vi "AngleStats_AngleAdd.vi"(6 "Row":i32, 10 "B":T1, 11 "A":T1) -> (3 "Result":T1)   [LabVIEW 2019, in "Trajectory_Library.lvlib"]
doc: "Creates a new LINEAR SYSTEM data cluster with the specified values. \n\n\nInputs: \n - XXX -- XXX.\n\nOutputs:\n - XXX -- XXX."
uses:
  <vilib>/Analysis/Matrix/Datatypes/RealMatrix.ctl
  MathUtil_InputModulus.vi
  Trajectory_Library.lvlib
  <vilib>/Analysis/Matrix/NI_Matrix.lvlib
  <vilib>/Analysis/Matrix/Numeric/Add/Add - RM,RM.vi
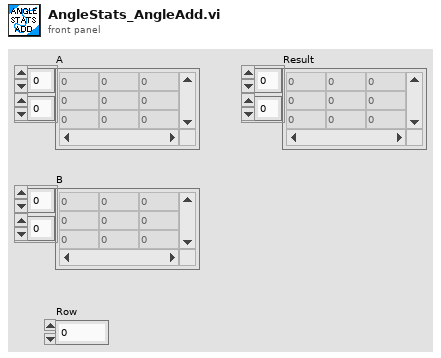
[diagram p1: front panel]
types:
  T1 = typedef "NI_Matrix.lvlib/RealMatrix.ctl" = dbl[][]
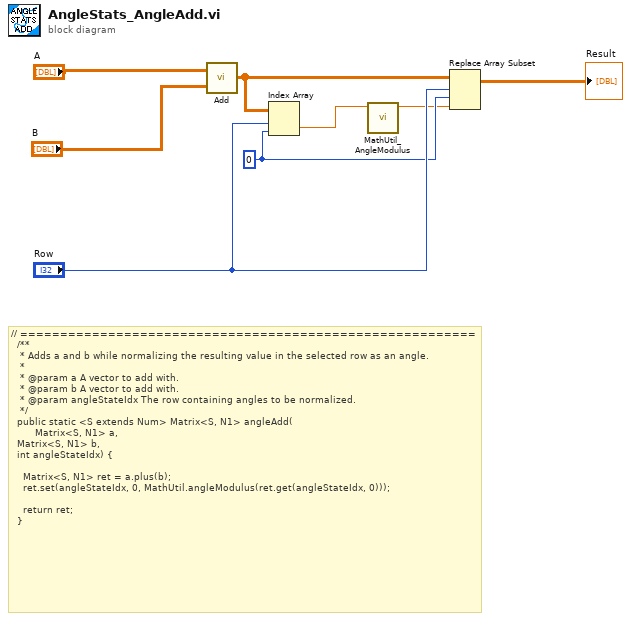
[diagram p0: block diagram]
diagram:
  w4 = 0 ("index (col)")
  # "// =========================================================\n  /**\n   * Adds a and b while normalizing the resulting value in the selected row as an angle.\n   *\n   * @param a A vector to add with.\n   * @param b A vector to add with.\n   * @param angleStateIdx The row containing angles to be normalized.\n   */\n  public static <S extends Num> Matrix<S, N1> angleAdd(\n      \t\tMatrix<S, N1> a, \n\t\tMatrix<S, N1> b, \n\t\tint angleStateIdx) {\n\n    Matrix<S, N1> ret = a.plus(b);\n    ret.set(angleStateIdx, 0, MathUtil.angleModulus(ret.get(angleStateIdx, 0)));\n\n    return ret;\n  }"
  n1 = call-poly <vilib>:"Add.vi"("Real Matrix B"="B", "Real Matrix A"="A") -> ("A + B"=w6:T1)
  n2 = Index Array(array=w6, index (row)="Row", index (col)=w4) -> (element=w2:dbl)
  n3 = call "MathUtil_AngleModulus.vi"("InputAngle"=w2) -> ("ModulsAngle"=w1:dbl)  [unwired: 10 in]
  n4 = Replace Array Subset(array=w6, new element=w1, index (row)="Row", index (col)=w4) -> (→"Result":T1)
